vi "HEAD.vi"(6 "timeout":i32=10000, 8 "error in":errorcluster, 10 "url":string, 11 "session in":refnum<class "Session.lvclass">) -> (0 "error out":errorcluster, 2 "headers":string, 3 "session out":refnum<class "Session.lvclass">, 4 "status code":u32)   [LabVIEW 2024, in "lib_NI_Advanced HTTP Client.lvlib" / "Session.lvclass"]
doc: "Sends a web request that returns headers from a server, web page, or web service. This VI uses the HEAD HTTP method. This VI does not submit any data to the server or receive body data. The minimal data exchange makes the HEAD VI useful for testing the validity of a URL."
uses:
  Session.lvclass
  Session.lvclass/Session.ctl
  lvwebclient_64.dll
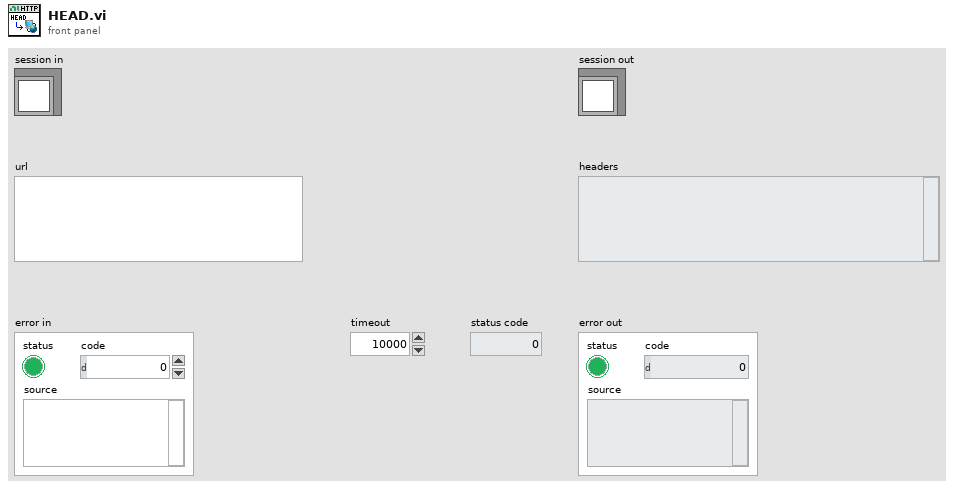
[diagram p1: front panel]
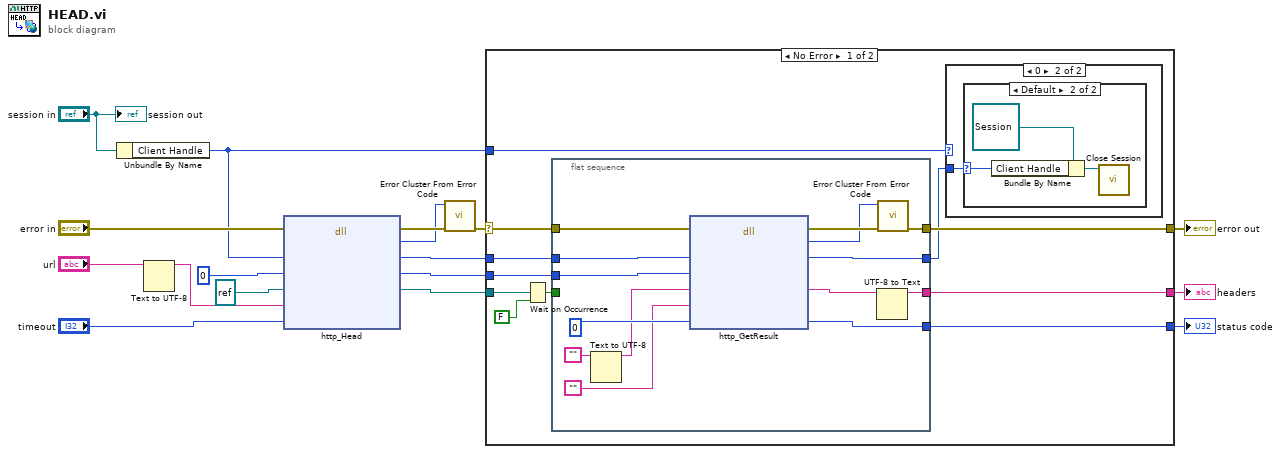
[diagram p0: block diagram]
diagram:
  n1 = Unbundle By Name("session in") -> ("Client Handle"=w8:u32)
  n2 = Text to UTF-8(11:"url") -> (3:w5:string)  [unwired: 2 in, 1 out]
  n3 = dll-call lib="C:/Program Files/National Instruments/LabVIEW 2024/vi.lib/NI/Advanced HTTP Client/lvwebclient_*.*" fn="http_Head"(error in="error in", "handle"=w8, "request"=u32 0, "completeOccurrence"=refnum<k4> refnum ("occurrence"), "url"=w5, "timeout"="timeout") -> (error out=w10:errorcluster, "return"=w9:i32, "handle"=w3:u32, "request"=w2:u32, "completeOccurrence"=w1:refnum<k4>)  [unwired: 4 in, 1 out]
  n4 = call "Error Cluster From Error Code.vi"("error in (no error)"=w10, "error code (0)"=w9) -> ("error out"=w17:errorcluster)  [unwired: 7 in]
  n5 = case shown="No Error" w17 {
    selector: w17 -> [w26 w47]
    tunnel: w1 -> [w28 _]
    tunnel: w3 -> [w25 _]
    tunnel: w2 -> [w24 _]
    tunnel: [w23 _] -> w14
    tunnel: [w22 _] -> w13
    tunnel: [w21 w47] -> w12
    tunnel: w8 -> [w20 _]
    frame No Error {
      n6 = Wait on Occurrence(1:FALSE, 2:w28) -> (0:w27:bool)  [unwired: 1 in]
      n7 = flat-sequence {
        tunnel: w27 -> [_]
        tunnel: w26 -> [w46]
        tunnel: w25 -> [w45]
        tunnel: w24 -> [w44]
        tunnel: [w42] -> w23
        tunnel: [w38] -> w22
        tunnel: [w37] -> w21
        tunnel: [w36] -> w19
        frame #0 {
          n8 = Text to UTF-8(11:"") -> (3:w34:string)  [unwired: 2 in, 1 out]
          n9 = dll-call lib="C:/Program Files/National Instruments/LabVIEW 2024/vi.lib/NI/Advanced HTTP Client/lvwebclient_*.*" fn="http_GetResult"(error in=w46, "handle"=w45, "request"=w44, "returnHeader"=w34, "returnBody"="", "httpStatus"=u32 0) -> (error out=w41:errorcluster, "return"=w40:i32, "handle"=w36:u32, "returnHeader"=w39:string, "httpStatus"=w42:u32)  [unwired: 4 in, 1 out]
          n10 = UTF-8 to Text(11:w39) -> (3:w38:string)  [unwired: 2 in, 1 out]
          n11 = call "Error Cluster From Error Code.vi"("error in (no error)"=w41, "error code (0)"=w40) -> ("error out"=w37:errorcluster)  [unwired: 7 in]
        }
      }
      n12 = case shown="0" w20 {
        tunnel: w19 -> [_ w29]
        frame Default {
        }
        frame 0 {
          n13 = case shown="Default" w29 {
            selector: w29 -> [_ w32]
            frame 0 {
            }
            frame Default {
              n14 = Bundle By Name(cluster=refnum<class "Session.lvclass"> refnum ("NI_Advanced HTTP Client.lvlib:Session.lvclass"), "Client Handle"=w32) -> (w31:refnum<class "Session.lvclass">)
              n15 = call "Close Session.vi"("session"=w31) -> ()  [unwired: 10 in, 1 out]
            }
          }
        }
      }
    }
    frame Error {
    }
  }
  "error out" <- w12
  "headers" <- w13
  "status code" <- w14
  "session out" <- "session in"
